vi "Destroy.vi"(8 "error in (no error)":errorcluster, 11 "CIF_NIChn_FIFO_DAQ in":refnum<class "CIF_NIChn_DAQ_Base.lvclass">) -> (0 "error out":errorcluster, 3 "CIF_NIChn_FIFO_DAQ out":refnum<class "CIF_NIChn_DAQ_Base.lvclass">)   [LabVIEW 2021, in "CIF_NIChn_DAQ_Base.lvclass"]
uses:
  CIF_NIChn_DAQ_Base.lvclass
  D:/dev/Packages/Channel_Manager/src/CIF_NIChn/NIChn/CIF_NIChn.lvclass
  D:/dev/Packages/Channel_Manager/src/CIFChannels/CIFChannels.lvclass
  NIChn/CIF_NIChn.lvclass/CIF_NIChn.ctl
  CIFChannels/CIFChannels.lvclass/CIFChannels.ctl
  CIF_NIChn_DAQ_Base.lvclass/CIF_NIChn_DAQ_Base.ctl
  Typedef/Datatype Waveform Channel.ctl
  <vilib>/CIF Foundation/CIF Channels/CIFChannels/SubVIs/CIFServices Fill In Error Info Ex.vi
  <vilib>/CIF Foundation/CIF Channels/CIFChannels/SubVIs/Get dll Path.vi
  <vilib>/CIF Foundation/CIF Utilities/Errors/Append Error Location.vi
  NIChn/CIF_NIChn.lvclass
  <vilib>/CIF Foundation/CIF Channels/CIFChannels/CIFChannelCore.lvlib
  CIFChannels/CIFChannels.lvclass
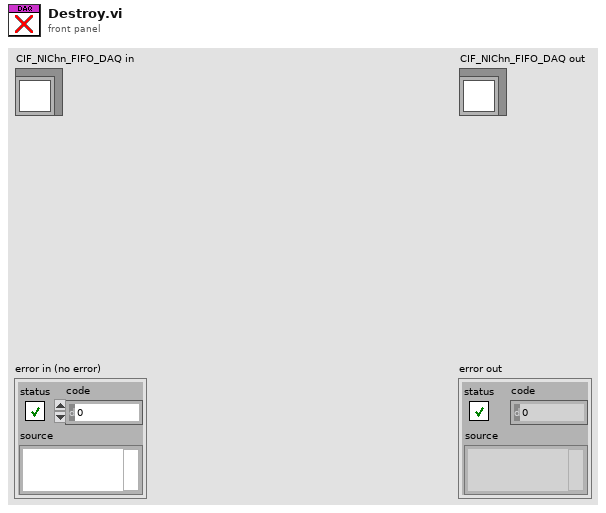
[diagram p1: front panel]
types:
  T1 = typedef "CIFChannels.lvclass/Direction.ctl" = enum16{"Publisher", "Subscriber"}
  T2 = typedef "ChannelCommon.lvlib/Datatype Waveform.ctl" = cluster{"measurement":dbl[], "dT":dbl, "Timestamp":i64, "Read Lock":bool}
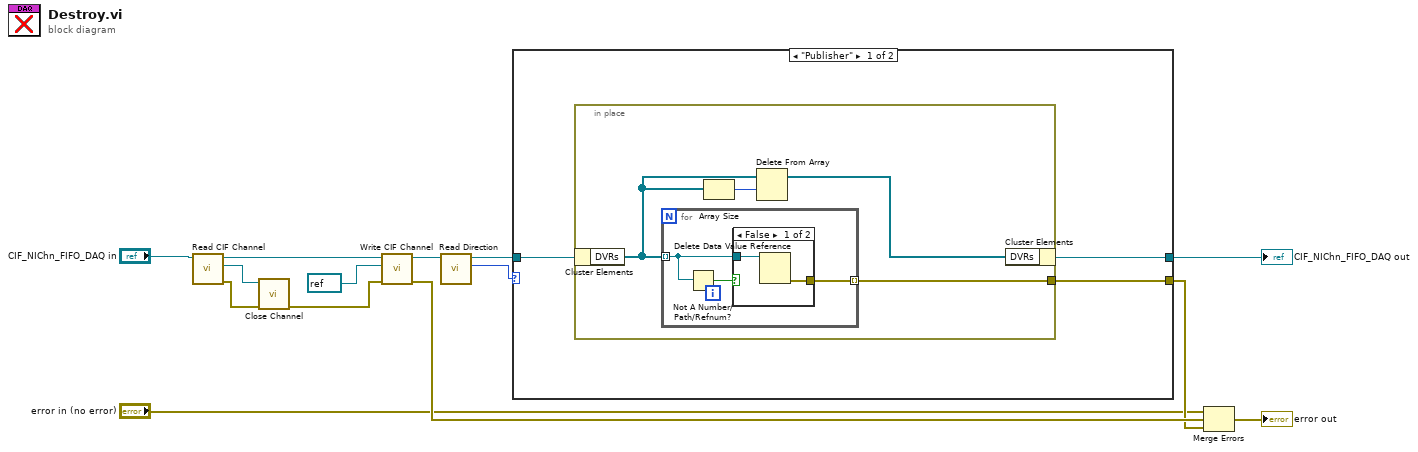
[diagram p0: block diagram]
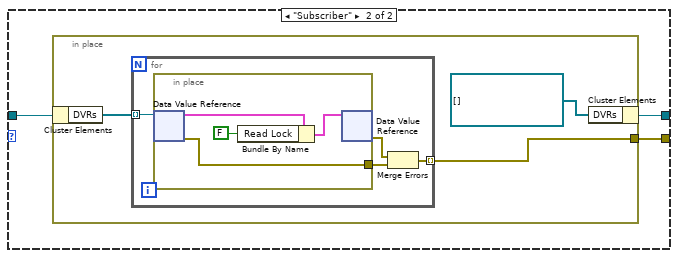
[diagram p3: hidden frame]
diagram:
  n1 = call "Read CIF Channel.vi"("CIFTag in"="CIF_NIChn_FIFO_DAQ in") -> ("error out"=w10:errorcluster, "CIF Channel"=w14:refnum<k21>, "CIFTag out"=w12:refnum<class "CIF_NIChn_DAQ_Base.lvclass">)  [unwired: 8 in]
  n2 = call <vilib>:"Close Channel.vi"("error in"=w10, "CIF Channel"=w14) -> ("error out"=w11:errorcluster)  [unwired: 9 in]
  n3 = call "Write CIF Channel.vi"("error in (no error)"=w11, "CIF Channel"=refnum<k21> refnum, "CIFTag in"=w12) -> ("error out"=w6:errorcluster, "CIFTag out"=w9:refnum<class "CIF_NIChn_DAQ_Base.lvclass">)  [unwired: 7 in]
  n4 = call "Read Direction.vi"("CIFChannels in"=w9) -> ("Direction"=w8:T1, "CIFChannels out"=w7:refnum<class "CIF_NIChn_DAQ_Base.lvclass">)  [unwired: 8 in, 1 out]
  n5 = case shown="\"Publisher\"" w8 {
    tunnel: [w17 w29] -> w1
    tunnel: w7 -> [w16 w28]
    tunnel: [w15 w27] -> w5
    frame "Publisher" {
      n6 = in-place {
        in-place-border: [w21] -> w15
        n7 = in-place-cluster #1(w16) -> ("DVRs"=w20:refnum<data-value>[])
        n8 = for {
          tunnel: w20 -> [w23] mode=indexing
          tunnel: [w24] -> w21 mode=indexing
          n9 = Not A Number/Path/Refnum?(number/path/refnum=w23) -> (NaN/Path/Refnum?=w22:bool)
          n10 = case shown="False" w22 {
            tunnel: [w26 _] -> w24
            tunnel: w23 -> [w25 _]
            frame False {
              n11 = Delete Data Value Reference(data value reference=w25) -> (error out=w26:errorcluster)  [unwired: 1 in, 1 out]
            }
            frame True {
            }
          }
        }
        n12 = Array Size(array=w20) -> (size(s)=w19:i32)
        n13 = Delete From Array(array=w20, length=w19) -> (array with subset deleted=w18:refnum<data-value>[])  [unwired: 1 in, 1 out]
        n14 = in-place-cluster #1("DVRs"=w18) -> (w17:refnum<class "CIF_NIChn_DAQ_Base.lvclass">)
      }
    }
    frame "Subscriber" {
      n15 = in-place {
        in-place-border: [w30] -> w27
        n16 = in-place-cluster #2(w28) -> ("DVRs"=w31:refnum<data-value>[])
        n17 = for {
          tunnel: w31 -> [w36] mode=indexing
          tunnel: [w33] -> w30 mode=indexing
          n18 = in-place {
            in-place-border: [w40] -> w35
            n19 = in-place-dvr #3(w36) -> (w39:T2, w40:errorcluster)
            n20 = Bundle By Name(cluster=w39, "Read Lock"=FALSE) -> (w38:T2)
            n21 = in-place-dvr #3(w38) -> (w34:errorcluster)  [unwired: 1 out]
          }
          n22 = Merge Errors(w34, w35) -> (w33:errorcluster)
        }
        n23 = in-place-cluster #2("DVRs"=refnum<data-value>[] []) -> (w29:refnum<class "CIF_NIChn_DAQ_Base.lvclass">)
      }
    }
  }
  "CIF_NIChn_FIFO_DAQ out" <- w1
  n24 = Merge Errors("error in (no error)", w6, w5) -> (→"error out":errorcluster)
